vi "AM Save SP Data Pk2Pk.vi"(8 "error in (no error)":errorcluster, 11 "Data Queue in":refnum<queue>) -> (0 "error out":errorcluster, 3 "Mean Data":dbl[](array[numeric]))   [LabVIEW 2020, in "Motion.lvlib"]
uses:
  Motion.lvlib
  support/PCT FGV CMD.ctl
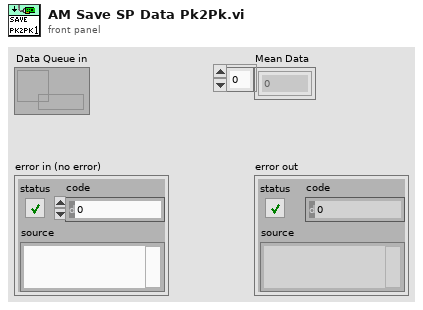
[diagram p1: front panel]
types:
  T1 = typedef "PCT FGV CMD.ctl" = enum16{"INIT", "GET", "SET"}
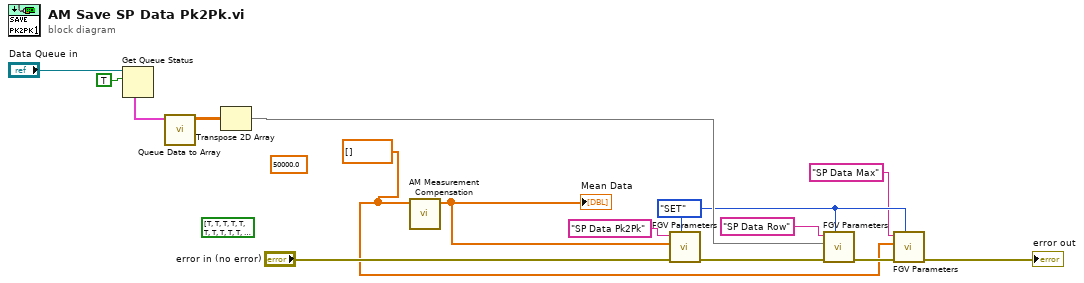
[diagram p0: block diagram]
diagram:
  w1 = dbl[] [] ("Mean Data")
  w4 = PCT_FGV_CMD."SET" ("CMD")
  (unwired) bool[] [TRUE, TRUE, TRUE, TRUE, TRUE, TRUE, TRUE, TRUE, TRUE, TRUE, TRUE, TRUE, TRUE, TRUE, TRUE, TRUE, TRUE, TRUE, TRUE, TRUE, TRUE, TRUE, TRUE, TRUE, TRUE, TRUE, TRUE, TRUE, TRUE, TRUE, TRUE, TRUE, TRUE, TRUE, TRUE, TRUE, TRUE, TRUE, TRUE, TRUE, TRUE, TRUE, TRUE, TRUE, TRUE, TRUE, TRUE, TRUE, TRUE, TRUE, TRUE, TRUE, TRUE, TRUE, TRUE, TRUE, TRUE, TRUE, TRUE, TRUE, TRUE, TRUE, TRUE, TRUE, TRUE, TRUE, TRUE, TRUE, TRUE, TRUE, TRUE, TRUE, TRUE, TRUE, TRUE, TRUE, TRUE, TRUE, TRUE, TRUE]
  (unwired) 50000.0 ("Criteria")
  n1 = Get Queue Status(queue="Data Queue in", return elements? (F)=TRUE) -> (elements=w10:cluster{"register values":dbl[][]}[])  [unwired: 1 in, 7 out]
  n2 = call "Queue Data to Array.vi"("elements"=w10) -> ("Array"=w12:dbl[][])  [unwired: 10 in]
  n3 = Transpose 2D Array(2D array=w12) -> (transposed array=w7:dbl[][])
  n4 = call "AM Measurement Compensation.vi"("Mean Data in"=w1) -> ("Mean Data Compensated out"=w2:dbl[])  [unwired: 10 in]
  "Mean Data" <- w2
  n5 = call "FGV Parameters.vi"("CMD"=w4, "error in (no error)"="error in (no error)", "input"=w2, "Key"="SP Data Pk2Pk") -> ("error out"=w9:errorcluster)  [unwired: 5 in, 2 out]
  n6 = call "FGV Parameters.vi"("CMD"=w4, "error in (no error)"=w9, "input"=w7, "Key"="SP Data Row") -> ("error out"=w6:errorcluster)  [unwired: 5 in, 2 out]
  n7 = call "FGV Parameters.vi"("CMD"=w4, "error in (no error)"=w6, "input"=w1, "Key"="SP Data Max") -> ("error out"=→"error out":errorcluster)  [unwired: 5 in, 2 out]
